vi "GetSource.vi"(6 "error in":errorcluster, 9 "Tunnel in":refnum<class "FlatSequenceInnerTunnel.lvclass">) -> (0 "error out":errorcluster, 3 "Tunnel out":refnum<class "FlatSequenceInnerTunnel.lvclass">, 4 "name":string)   [LabVIEW 2014, in "Raspberry Pi Compatible Compiler for LabVIEW.lvlib" / "FlatSequenceInnerTunnel.lvclass"]
uses:
  FlatSequenceInnerTunnel.lvclass
  FlatSequenceInnerTunnel.lvclass/FlatSequenceInnerTunnel.ctl
  Terminal/Terminal.lvclass
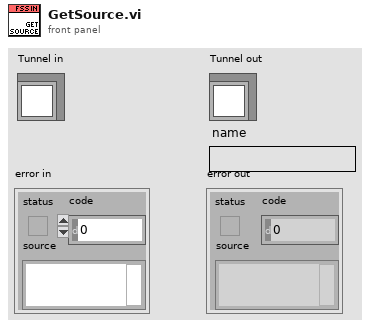
[diagram p1: front panel]
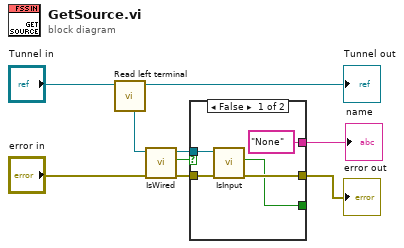
[diagram p0: block diagram]
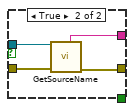
[diagram p2: hidden frame]
diagram:
  n1 = call "Read left terminal.vi"("FlatSequenceInnerTunnel in"="Tunnel in") -> ("FlatSequenceInnerTunnel out"=→"Tunnel out":refnum<class "FlatSequenceInnerTunnel.lvclass">, "left terminal"=w5:refnum<class "Terminal.lvclass">)  [unwired: 7 in]
  n2 = call "IsWired.vi"("error in"="error in", "Terminal in"=w5) -> ("error out"=w1:errorcluster, "wired"=w3:bool, "Terminal out"=w2:refnum<class "Terminal.lvclass">)  [unwired: 5 in]
  n3 = case shown="False" w3 {
    tunnel: ["None" ("name") w16] -> w7
    tunnel: [w11 w15] -> w6
    tunnel: w2 -> [w12 w18]
    tunnel: w1 -> [w13 w17]
    tunnel: [w10 _] -> _
    frame False {
      n4 = call-dynamic "IsInput.vi"("error in"=w13, "Terminal in"=w12) -> ("error out"=w11:errorcluster, "input"=w10:bool)  [unwired: 5 in, 1 out]
    }
    frame True {
      n5 = call "GetSourceName.vi"("error in"=w17, "Terminal in"=w18) -> ("error out"=w15:errorcluster, "source"=w16:string)  [unwired: 5 in, 1 out]
    }
  }
  "error out" <- w6
  "name" <- w7
